vi "NewStepTypeDialog.vi"() -> (1 "Step Name Out":string, 2 "Step Type Out":T1, 3 "Cancel?":bool)   [LabVIEW 2014, in "Project.lvclass"]
uses:
  Project.lvclass
  StepData/Control/StepTypeEnum.ctl
  StepData/StepData.lvclass
panel:
  in  "Step Type":T1
  in  "Step Name":string
  in  "Cancel":bool
  in  "OK":bool
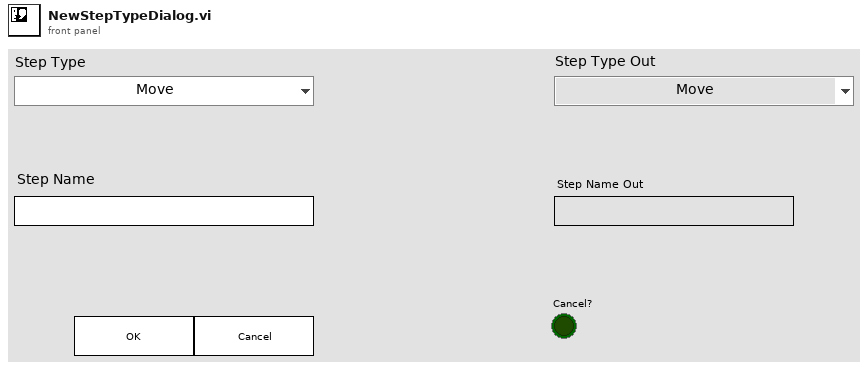
[diagram p1: front panel]
types:
  T1 = typedef "StepData.lvclass/StepTypeEnum.ctl" = enum16{"Move", "Measure"}
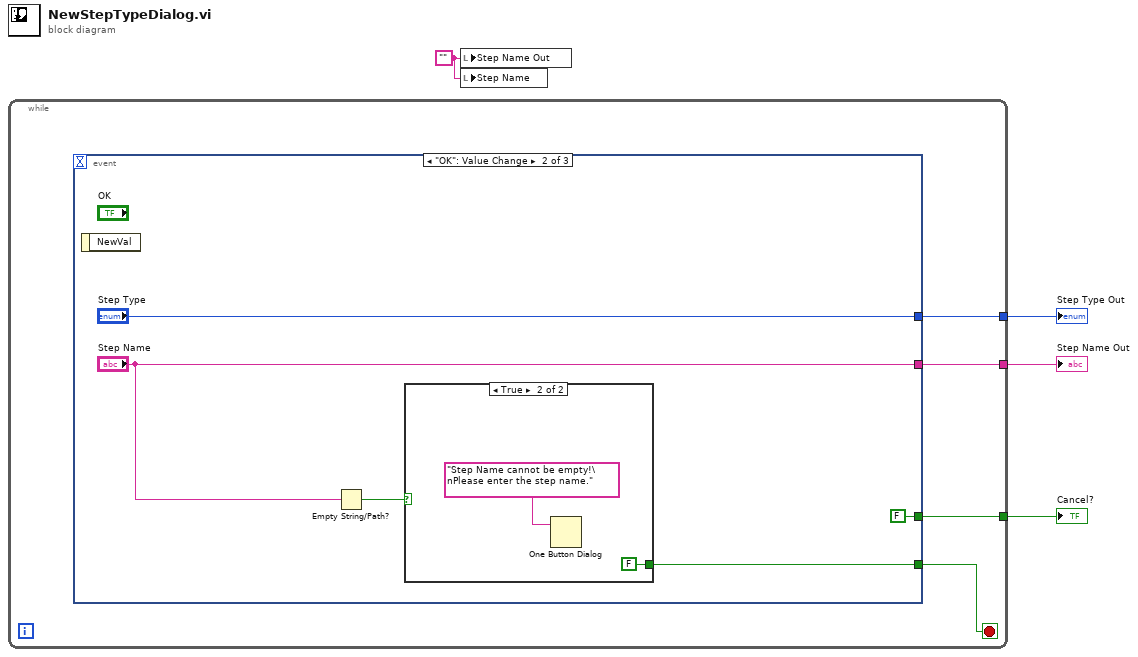
[diagram p0: block diagram]
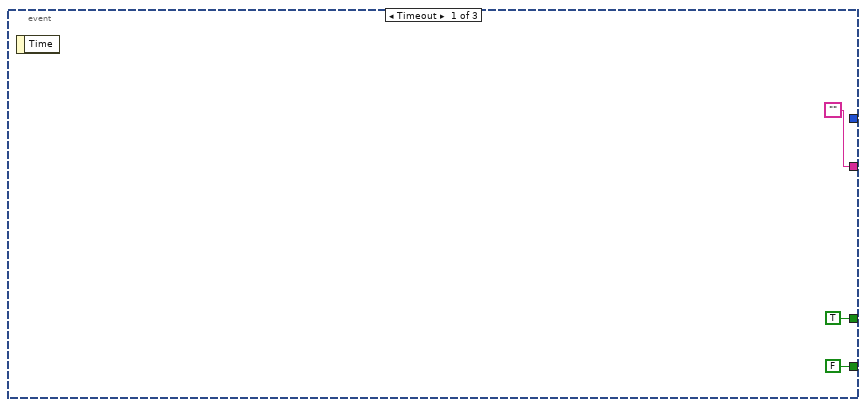
[diagram p2: hidden frame]
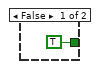
[diagram p3: hidden frame]
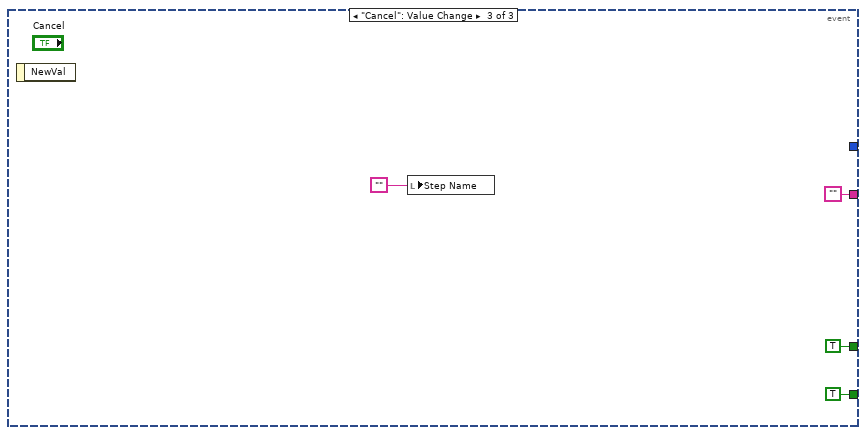
[diagram p4: hidden frame]
diagram:
  w1 = "" ("Step Name Out")
  n1 = while {
    tunnel: [w7] -> w4
    tunnel: [w6] -> w3
    tunnel: [w5] -> w2
    stop <- w8 stop-if-true
    n2 = event shown="[1] \"OK\": Value Change" {
      selector: _ -> [_ _ _]
      dyn-events: _ -> [_ _ _]
      timeout: _ -> [_ _ _]
      tunnel: [FALSE w13 TRUE] -> w8
      tunnel: [TRUE FALSE TRUE] -> w7
      tunnel: ["" ("Step Name") "Step Name" "" ("Step Name")] -> w6
      tunnel: [_ "Step Type" _] -> w5
      event Timeout {
        n3 = event-data() -> ()  [unwired: 1 in, 1 out]
      }
      event "OK": Value Change {
        n4 = event-data() -> ()  [unwired: 1 in, 1 out]
        n5 = Empty String/Path?(string/path="Step Name") -> (empty?=w15:bool)
        n6 = case shown="True" w15 {
          tunnel: [TRUE FALSE] -> w13
          frame False {
          }
          frame True {
            n7 = One Button Dialog(message="Step Name cannot be empty!\nPlease enter the step name.") -> ()  [unwired: 1 in, 1 out]
          }
        }
      }
      event "Cancel": Value Change {
        n8 = event-data() -> ()  [unwired: 1 in, 1 out]
        n9 = local write "Step Name"("" ("Step Name Out")) -> ()
      }
    }
  }
  "Cancel?" <- w4
  "Step Name Out" <- w3
  "Step Type Out" <- w2
  n10 = local write "Step Name Out"(w1) -> ()
  n11 = local write "Step Name"(w1) -> ()
